vi "Initialize.vi"(8 "Error In":errorcluster) -> (0 "Error Out":errorcluster, 3 "Central Message Handler":refnum<class "Central Message Handler.lvclass">)   [LabVIEW 2021, in "Central Message Handler.lvclass"]
uses:
  Central Message Handler.lvclass
  Controls/Message.ctl
  Private/Controls/Data.ctl
  Process/Public/Controls/Process Message.ctl
  Process/Process.lvclass
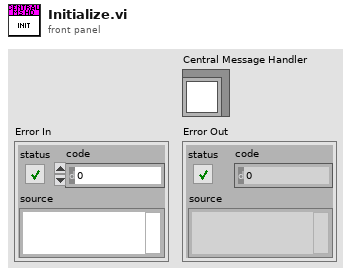
[diagram p1: front panel]
types:
  T1 = typedef "Central Message Handler.lvclass/Data.ctl" = cluster{"Central Message Queue":refnum<queue>, "Processes Queues Map":map{string, refnum<queue>}}
  T2 = typedef "Central Message Handler.lvclass/Message.ctl" = cluster{"Command":string, "Data":variant, "Receiver":string}
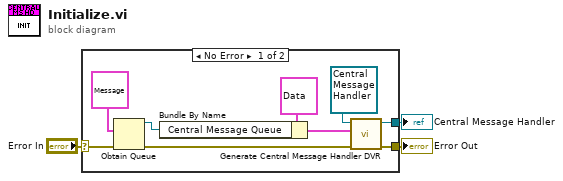
[diagram p0: block diagram]
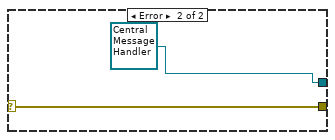
[diagram p2: hidden frame]
diagram:
  n1 = case shown="No Error" "Error In" {
    selector: "Error In" -> [w11 w14]
    tunnel: [w9 w14] -> w2
    tunnel: [w8 refnum<class "Central Message Handler.lvclass"> refnum ("Central Message Handler Out")] -> w1
    frame No Error {
      n2 = Obtain Queue(element data type=T2 {"Command"="", "Data"=variant, "Receiver"=""} ("Message"), error in (no error)=w11) -> (queue out=w6:refnum<queue>, error out=w4:errorcluster)  [unwired: 3 in, 1 out]
      n3 = Bundle By Name(cluster=T1 {"Central Message Queue"=refnum, "Processes Queues Map"={}} ("Data"), "Central Message Queue"=w6) -> (w5:T1)
      n4 = call "Generate Central Message Handler DVR.vi"("Error In"=w4, "Data"=w5, "Central Message Handler In"=refnum<class "Central Message Handler.lvclass"> refnum) -> ("Error Out"=w9:errorcluster, "Central Message Handler Out"=w8:refnum<class "Central Message Handler.lvclass">)  [unwired: 7 in]
    }
    frame Error {
    }
  }
  "Error Out" <- w2
  "Central Message Handler" <- w1
